vi "add_subpattern_to_raps_points.vi"(8 "error in (no error)":errorcluster, 9 "subpattern delty y":i32[](array[numeric]), 10 "subpattern delta x":i32[](array[numeric]), 11 "TrajectoryMH100122AODRAPS in":refnum<class "TrajectoryMH100122AODRAPS.lvclass">) -> (0 "error out":errorcluster, 3 "TrajectoryMH100122AODRAPS out":refnum<class "TrajectoryMH100122AODRAPS.lvclass">)   [LabVIEW 2010, in "TrajectoryMH100122AODRAPS.lvclass"]
uses:
  TrajectoryMH100122AODRAPS.lvclass
  TrajectoryMH100122AODRAPS.lvclass/TrajectoryMH100122AODRAPS.ctl
panel:
  out "RAPS points cluster.x array 2":u16[](array[numeric])
  out "RAPS points cluster.x array":u16[](array[numeric])
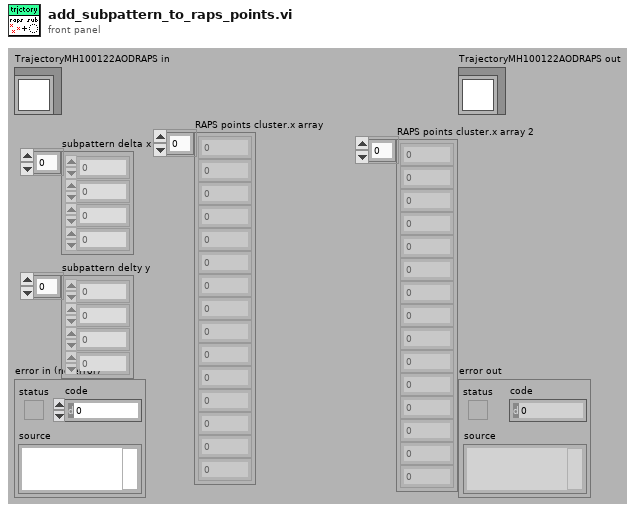
[diagram p1: front panel]
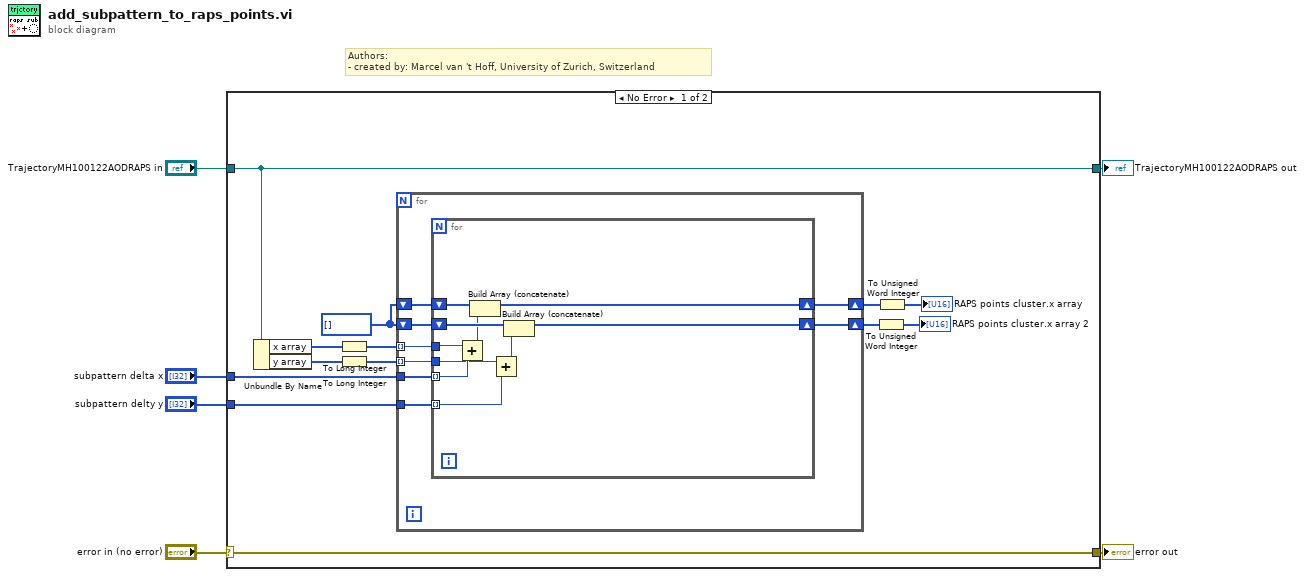
[diagram p0: block diagram]
diagram:
  # "Authors: \n- created by: Marcel van 't Hoff, University of Zurich, Switzerland"
  n1 = case shown="No Error" "error in (no error)" {
    selector: "error in (no error)" -> [w19 w39]
    tunnel: [w19 w39] -> w5
    tunnel: [w18 w38] -> w3
    tunnel: "TrajectoryMH100122AODRAPS in" -> [w18 w38]
    tunnel: "subpattern delta x" -> [w15 _]
    tunnel: "subpattern delty y" -> [w14 _]
    frame No Error {
      w13 = i32[] [] ("RAPS points cluster.x array")
      n2 = Unbundle By Name(w18) -> ("x array"=w17:u16[], "y array"=w16:u16[])
      n3 = To Long Integer(number=w17) -> (32bit integer=w11:i32[])
      n4 = To Long Integer(number=w16) -> (32bit integer=w10:i32[])
      n5 = for {
        tunnel: w11 -> [w21] mode=indexing
        tunnel: w10 -> [w20] mode=indexing
        shift-right: [w23] -> w12
        shift-left: w13 -> [w25]
        tunnel: w14 -> [w26]
        tunnel: w15 -> [w27]
        shift-right: [w22] -> w9
        shift-left: w13 -> [w24]
        n6 = for {
          tunnel: w27 -> [w32] mode=indexing
          tunnel: w26 -> [w29] mode=indexing
          tunnel: w21 -> [w33]
          tunnel: w20 -> [w30]
          shift-right: [w35] -> w22
          shift-left: w24 -> [w36]
          shift-right: [w34] -> w23
          shift-left: w25 -> [w37]
          n7 = Add(x=w33, y=w32) -> (x+y=w31:i32)
          n8 = Build Array (concatenate)(w36, w31) -> (w35:i32[])
          n9 = Add(x=w30, y=w29) -> (x+y=w28:i32)
          n10 = Build Array (concatenate)(w37, w28) -> (w34:i32[])
        }
      }
      n11 = To Unsigned Word Integer(number=w12) -> (unsigned 16bit integer=→"RAPS points cluster.x array 2":u16[])
      n12 = To Unsigned Word Integer(number=w9) -> (unsigned 16bit integer=→"RAPS points cluster.x array":u16[])
    }
    frame Error {
    }
  }
  "error out" <- w5
  "TrajectoryMH100122AODRAPS out" <- w3
